vi "Defaults.vi"(8 "error in (no error)":errorcluster, 11 "Sim DiscreteIO in":refnum<class "Sim DiscreteIO.lvclass">) -> (0 "error out":errorcluster, 3 "Sim DiscreteIO out":refnum<class "Sim DiscreteIO.lvclass">)   [LabVIEW 2021, in "Sim DiscreteIO.lvclass"]
uses:
  Sim DiscreteIO.lvclass
  C:/Program Files (x86)/National Instruments/LabVIEW 2021/user.lib/S2 Labs/Module Framework/Modules/Base/Module.lvclass
  Sim DiscreteIO.lvclass/Sim DiscreteIO.ctl
  <userlib>/S2 Labs/Module Framework/Modules/Base/Module.lvclass/Module.ctl
  Accessors/Write ch_labels.vi
  Accessors/Write ch_alias.vi
  Accessors/Write ch_units.vi
  <userlib>/S2 Labs/Module Framework/Modules/Base/Write Timeout (ms).vi
  <userlib>/S2 Labs/Module Framework/Modules/Base/Module.lvclass
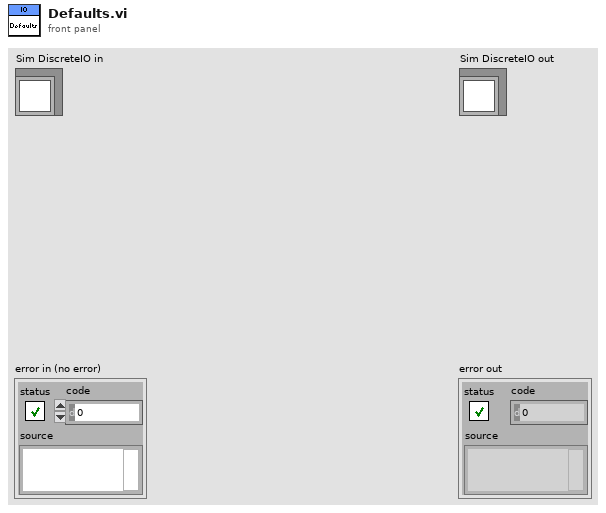
[diagram p1: front panel]
types:
  T1 = cluster{"label":string, "alias":string, "unit":string}[]
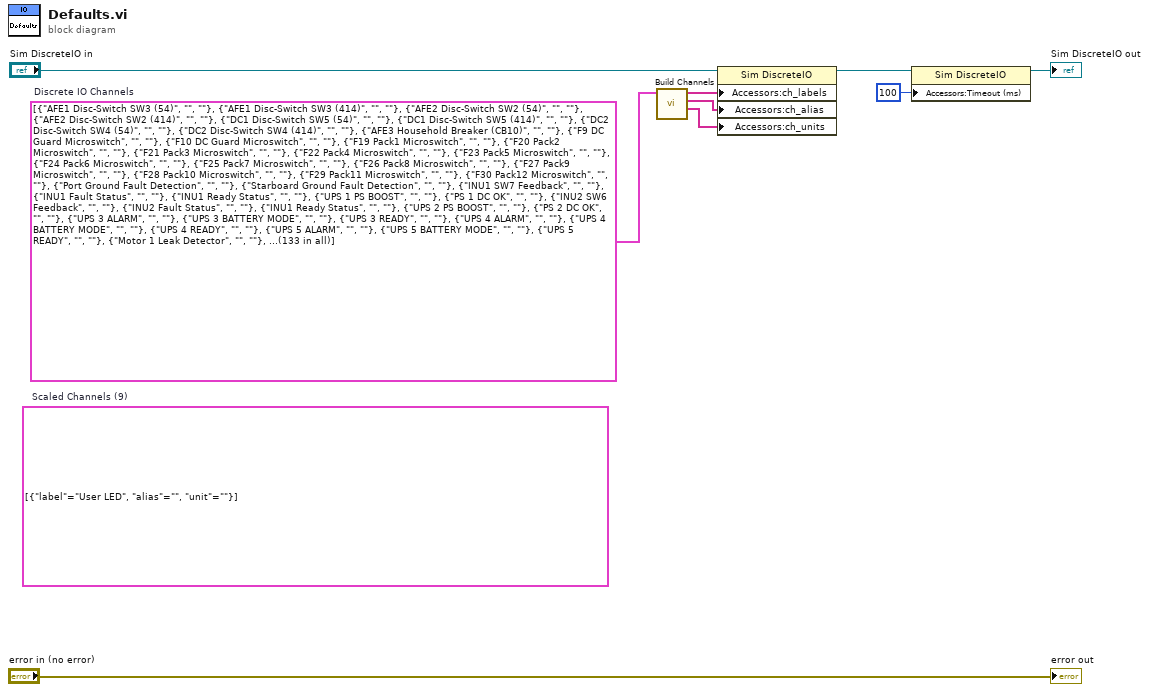
[diagram p0: block diagram]
diagram:
  (unwired) T1 [{"label"="User LED", "alias"="", "unit"=""}]  # Scaled Channels (9)
  w1 = T1 [{"label"="AFE1 Disc-Switch SW3 (54)", "alias"="", "unit"=""}, {"label"="AFE1 Disc-Switch SW3 (414)", "alias"="", "unit"=""}, {"label"="AFE2 Disc-Switch SW2 (54)", "alias"="", "unit"=""}, {"label"="AFE2 Disc-Switch SW2 (414)", "alias"="", "unit"=""}, {"label"="DC1 Disc-Switch SW5 (54)", "alias"="", "unit"=""}, {"label"="DC1 Disc-Switch SW5 (414)", "alias"="", "unit"=""}, {"label"="DC2 Disc-Switch SW4 (54)", "alias"="", "unit"=""}, {"label"="DC2 Disc-Switch SW4 (414)", "alias"="", "unit"=""}, {"label"="AFE3 Household Breaker (CB10)", "alias"="", "unit"=""}, {"label"="F9 DC Guard Microswitch", "alias"="", "unit"=""}, {"label"="F10 DC Guard Microswitch", "alias"="", "unit"=""}, {"label"="F19 Pack1 Microswitch", "alias"="", "unit"=""}, {"label"="F20 Pack2 Microswitch", "alias"="", "unit"=""}, {"label"="F21 Pack3 Microswitch", "alias"="", "unit"=""}, {"label"="F22 Pack4 Microswitch", "alias"="", "unit"=""}, {"label"="F23 Pack5 Microswitch", "alias"="", "unit"=""}, {"label"="F24 Pack6 Microswitch", "alias"="", "unit"=""}, {"label"="F25 Pack7 Microswitch", "alias"="", "unit"=""}, {"label"="F26 Pack8 Microswitch", "alias"="", "unit"=""}, {"label"="F27 Pack9 Microswitch", "alias"="", "unit"=""}, {"label"="F28 Pack10 Microswitch", "alias"="", "unit"=""}, {"label"="F29 Pack11 Microswitch", "alias"="", "unit"=""}, {"label"="F30 Pack12 Microswitch", "alias"="", "unit"=""}, {"label"="Port Ground Fault Detection", "alias"="", "unit"=""}, {"label"="Starboard Ground Fault Detection", "alias"="", "unit"=""}, {"label"="INU1 SW7 Feedback", "alias"="", "unit"=""}, {"label"="INU1 Fault Status", "alias"="", "unit"=""}, {"label"="INU1 Ready Status", "alias"="", "unit"=""}, {"label"="UPS 1 PS BOOST", "alias"="", "unit"=""}, {"label"="PS 1 DC OK", "alias"="", "unit"=""}, {"label"="INU2 SW6 Feedback", "alias"="", "unit"=""}, {"label"="INU2 Fault Status", "alias"="", "unit"=""}, {"label"="INU1 Ready Status", "alias"="", "unit"=""}, {"label"="UPS 2 PS BOOST", "alias"="", "unit"=""}, {"label"="PS 2 DC OK", "alias"="", "unit"=""}, {"label"="UPS 3 ALARM", "alias"="", "unit"=""}, {"label"="UPS 3 BATTERY MODE", "alias"="", "unit"=""}, {"label"="UPS 3 READY", "alias"="", "unit"=""}, {"label"="UPS 4 ALARM", "alias"="", "unit"=""}, {"label"="UPS 4 BATTERY MODE", "alias"="", "unit"=""}, {"label"="UPS 4 READY", "alias"="", "unit"=""}, {"label"="UPS 5 ALARM", "alias"="", "unit"=""}, {"label"="UPS 5 BATTERY MODE", "alias"="", "unit"=""}, {"label"="UPS 5 READY", "alias"="", "unit"=""}, {"label"="Motor 1 Leak Detector", "alias"="", "unit"=""}, {"label"="Motor 1 Grease Feedback", "alias"="", "unit"=""}, {"label"="Motor 2 Leak Detector", "alias"="", "unit"=""}, {"label"="Motor 2 Grease Feedback", "alias"="", "unit"=""}, {"label"="Water Sensor Drip Sensors", "alias"="", "unit"=""}, {"label"="Spare S2 DI17", "alias"="", "unit"=""}, {"label"="Spare S2 DI18", "alias"="", "unit"=""}, {"label"="Battery Array 1 E-Stop Indicator", "alias"="", "unit"=""}, {"label"="Battery Array 2 E-Stop Indicator", "alias"="", "unit"=""}, {"label"="SS Ahead Signal", "alias"="", "unit"=""}, {"label"="SS Astern Signal", "alias"="", "unit"=""}, {"label"="PS Ahead Signal", "alias"="", "unit"=""}, {"label"="PS Astern Signal", "alias"="", "unit"=""}, {"label"="Port Coolant Level Sensor", "alias"="", "unit"=""}, {"label"="Starboard Coolant Level Sensor", "alias"="", "unit"=""}, {"label"="Motor 1 E-Stop Indicator", "alias"="", "unit"=""}, {"label"="Motor 2 E-Stop Indicator", "alias"="", "unit"=""}, {"label"="raw_Port Coolant Flowrate", "alias"="", "unit"="Hz"}, {"label"="raw_Starboard Coolant Flowrate", "alias"="", "unit"="Hz"}, {"label"="AFE1 Recycle Control Relay", "alias"="", "unit"=""}, {"label"="AFE2 Recycle Control Relay", "alias"="", "unit"=""}, {"label"="DC1 Recycle Control Relay", "alias"="", "unit"=""}, {"label"="DC2 Recycle Control Relay", "alias"="", "unit"=""}, {"label"="INU1 Recycle Control Relay", "alias"="", "unit"=""}, {"label"="INU2 Recycle Control Relay", "alias"="", "unit"=""}, {"label"="AFE3 Recycle Control Relay", "alias"="", "unit"=""}, {"label"="AFE1 Disc-Switch SW3 CLOSING COIL RELAY", "alias"="", "unit"=""}, {"label"="AFE1 Disc-Switch SW3  SHUNT COIL RELAY", "alias"="", "unit"=""}, {"label"="AFE2 Disc-Switch SW2 CLOSING COIL RELAY", "alias"="", "unit"=""}, {"label"="AFE2 Disc-Switch SW2  SHUNT COIL RELAY", "alias"="", "unit"=""}, {"label"="DC1 Disc-Switch SW5 CLOSING COIL RELAY", "alias"="", "unit"=""}, {"label"="DC1 Disc-Switch SW5  SHUNT COIL RELAY", "alias"="", "unit"=""}, {"label"="DC2 Disc-Switch SW4 CLOSING COIL RELAY", "alias"="", "unit"=""}, {"label"="DC2 Disc-Switch SW4  SHUNT COIL RELAY", "alias"="", "unit"=""}, {"label"="AFE1 Reset Control Relay", "alias"="", "unit"=""}, {"label"="AFE2 Reset Control Relay", "alias"="", "unit"=""}, {"label"="DC1 Reset Control Relay", "alias"="", "unit"=""}, {"label"="DC2 Reset Control Relay", "alias"="", "unit"=""}, {"label"="INU1 Reset Control Relay", "alias"="", "unit"=""}, {"label"="INU2 Reset Control Relay", "alias"="", "unit"=""}, {"label"="AFE3 Reset Control Relay", "alias"="", "unit"=""}, {"label"="INU1 Run Enable", "alias"="", "unit"=""}, {"label"="INU1 Pre-Charge Contactor", "alias"="", "unit"=""}, {"label"="INU1 Ahead Output Signal", "alias"="", "unit"=""}, {"label"="INU1 Astern Output Signal", "alias"="", "unit"=""}, {"label"="INU2 Run Enable", "alias"="", "unit"=""}, {"label"="INU2 Pre-Charge Contactor", "alias"="", "unit"=""}, {"label"="INU2 Ahead Output Signal", "alias"="", "unit"=""}, {"label"="INU2 Astern Output Signal", "alias"="", "unit"=""}, {"label"="BMS UPS REMOTE", "alias"="", "unit"=""}, {"label"="BMS UPS BAT-START", "alias"="", "unit"=""}, {"label"="Power Enclosure Red Indicating Light", "alias"="", "unit"=""}, {"label"="Power Enclosure Amber Indicating Light", "alias"="", "unit"=""}, {"label"="Power Enclosure Green Indicating Light", "alias"="", "unit"=""}, {"label"="Battery Array 1 E-Stop Safety Relay Start", "alias"="", "unit"=""}, {"label"="Battery Array 2 E-Stop Safety Relay Start", "alias"="", "unit"=""}, {"label"="Motor 1 Grease power", "alias"="", "unit"=""}, {"label"="Motor 1 Grease Pulse", "alias"="", "unit"=""}, {"label"="Motor 1 E-Stop Safety Relay Start", "alias"="", "unit"=""}, {"label"="Motor 2 Grease power", "alias"="", "unit"=""}, {"label"="Motor 2 Grease Pulse", "alias"="", "unit"=""}, {"label"="Motor 2 E-Stop Safety Relay Start", "alias"="", "unit"=""}, {"label"="Motor 1 Heater", "alias"="", "unit"=""}, {"label"="Motor 2 Heater", "alias"="", "unit"=""}, {"label"="Port Cooling Heaters 1", "alias"="", "unit"=""}, {"label"="Starboard Cooling Heaters 2", "alias"="", "unit"=""}, {"label"="DCG1 Start", "alias"="", "unit"=""}, {"label"="DCG2 Start", "alias"="", "unit"=""}, {"label"="INU1 Switch Open", "alias"="", "unit"=""}, {"label"="INU1 Switch Close", "alias"="", "unit"=""}, {"label"="INU2 Switch Open", "alias"="", "unit"=""}, {"label"="INU2 Switch Close", "alias"="", "unit"=""}, {"label"="DC1 Pre-Charge", "alias"="", "unit"=""}, {"label"="DC1 Breaker CB13 Closing Coil", "alias"="", "unit"=""}, {"label"="DC1 Breaker CB13 Shunt Open Coil", "alias"="", "unit"=""}, {"label"="DC2 Pre-Charge", "alias"="", "unit"=""}, {"label"="DC2 Breaker CB14 Closing Coil", "alias"="", "unit"=""}, {"label"="DC2 Breaker CB14 Shunt Open Coil", "alias"="", "unit"=""}, {"label"="raw_Throttle CMD Signal Port", "alias"="", "unit"="mA"}, {"label"="raw_Throttle CMD Signal Starboard", "alias"="", "unit"="mA"}, {"label"="raw_Port Cooling Pressure Trans", "alias"="", "unit"="mA"}, {"label"="raw_Starboard Cooling Pressure Trans", "alias"="", "unit"="mA"}, {"label"="raw_Port Coolant Temp Sensor", "alias"="", "unit"="mA"}, {"label"="raw_Starboard Coolant Temp Sensor", "alias"="", "unit"="mA"}, {"label"="raw_RTD Enclosure", "alias"="", "unit"="mA"}, {"label"="raw_RTD DC Guard 1 Filter", "alias"="", "unit"="mA"}, {"label"="raw_RTD DC Guard 2 Filter", "alias"="", "unit"="mA"}, {"label"="raw_Port INU1 Motor 1 Speed", "alias"="", "unit"="mA"}, {"label"="raw_Starboard INU2 Motor 2 Speed", "alias"="", "unit"="mA"}]  # Discrete IO Channels
  n1 = call <userlib>:"Build Channels.vi"("chs"=w1) -> ("ch_units"=w6:string[], "ch_alias"=w5:string[], "ch_labels"=w4:string[])  [unwired: 8 in]
  n2 = property class="Sim DiscreteIO"(reference="Sim DiscreteIO in", "Accessors:ch_labels"=w4, "Accessors:ch_alias"=w5, "Accessors:ch_units"=w6) -> (reference out=w2:refnum<class "Sim DiscreteIO.lvclass">)  [unwired: 1 in, 1 out]
  n3 = property class="Sim DiscreteIO"(reference=w2, "Accessors:Timeout (ms)"=100 ("Module:Timeout (ms)")) -> (reference out=→"Sim DiscreteIO out":refnum<class "Sim DiscreteIO.lvclass">)  [unwired: 1 in, 1 out]
  "error out" <- "error in (no error)"
